vi "NumIntegrate_Rkf45_Func_B1.vi"(11 "Index":i32) -> (3 "RKF45_B1":dbl)   [LabVIEW 2019, in "Trajectory_Library.lvlib"]
doc: "Internal function used by Rkdp_Impl.vi\n\nInputs:\n - Index -- Index into B1 array (must be 0 - 6 )\n\nOutputs:\n - B1 -- Value looked up by index."
uses:
  Trajectory_Library.lvlib
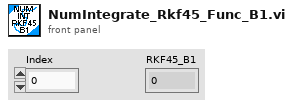
[diagram p1: front panel]
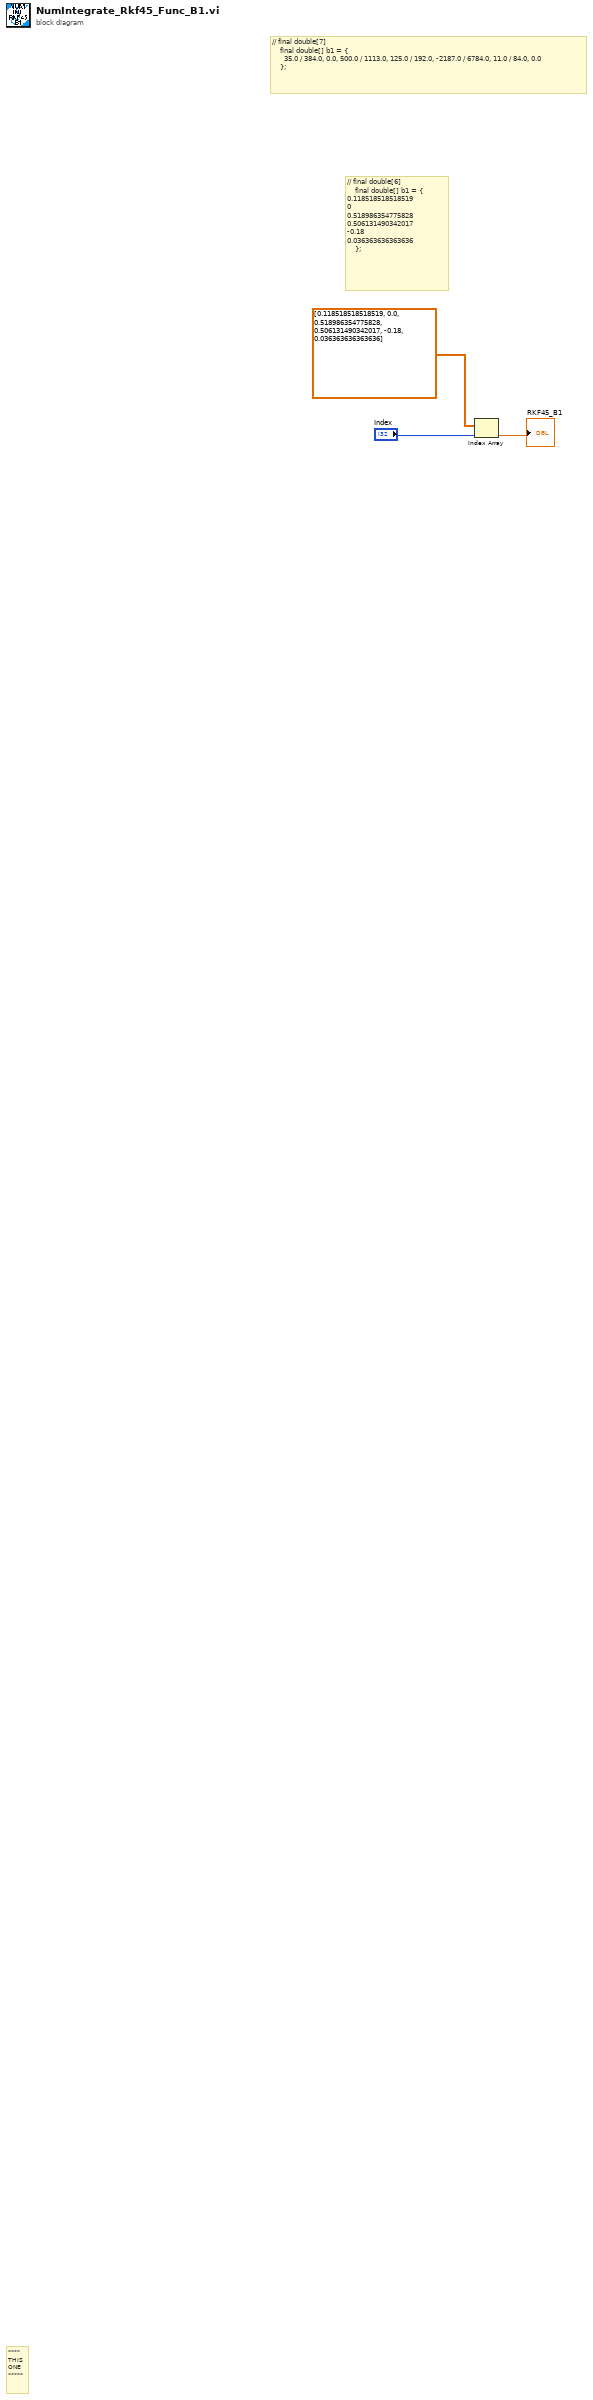
[diagram p0: block diagram]
diagram:
  # "// final double[6]\t\t\t\t\t\n    final double[] b1 = {\t\t\t\t\t\n0.118518518518519\t\n0\t\n0.518986354775828\t\n0.506131490342017\t\n-0.18\t\n0.036363636363636\n    };"
  # "// final double[7]\n    final double[] b1 = {\n      35.0 / 384.0, 0.0, 500.0 / 1113.0, 125.0 / 192.0, -2187.0 / 6784.0, 11.0 / 84.0, 0.0\n    };"
  # "****\nTHIS\nONE\n*****"
  n1 = Index Array(array=dbl[] [0.118518518518519, 0.0, 0.518986354775828, 0.506131490342017, -0.18, 0.036363636363636], index="Index") -> (element=→"RKF45_B1":dbl)
